vi "Check Target Internet Connection.vi"(8 "Error In":errorcluster, 11 "Install LV Data":T1={"SSH Session"=refnum, "Status Log"="", "Detailed Log"="", "Credentials"={"Hostname or IP"="192.168.7.2", "Username"="root", "Password"=""}, "Target Info"={"OS Version"="", "CPU"="", "Systemd Version"="", "Internet Access"=FALSE, "Device Type"=""}, "Reboot Required?"=FALSE}) -> (0 "Error Out":errorcluster, 3 "Install LV Data":T1={"SSH Session"=refnum, "Status Log"="", "Detailed Log"="", "Credentials"={"Hostname or IP"="192.168.7.2", "Username"="root", "Password"=""}, "Target Info"={"OS Version"="", "CPU"="", "Systemd Version"="", "Internet Access"=FALSE, "Device Type"=""}, "Reboot Required?"=FALSE})   [LabVIEW 2014, in "LMH-LINX.lvlib"]
uses:
  LMH-LINX.lvlib
  Install LV Data.ctl
  C:/github/makerhub/LINX/LabVIEW/vi.lib/MakerHub/LINX/Resources/Renci.SshNet.dll
  Resources/Renci.SshNet.dll
  Target Info.ctl
  <vilib>/regexp/Match Regular Expression.xnode
panel:
  out "Internet Connection?":bool
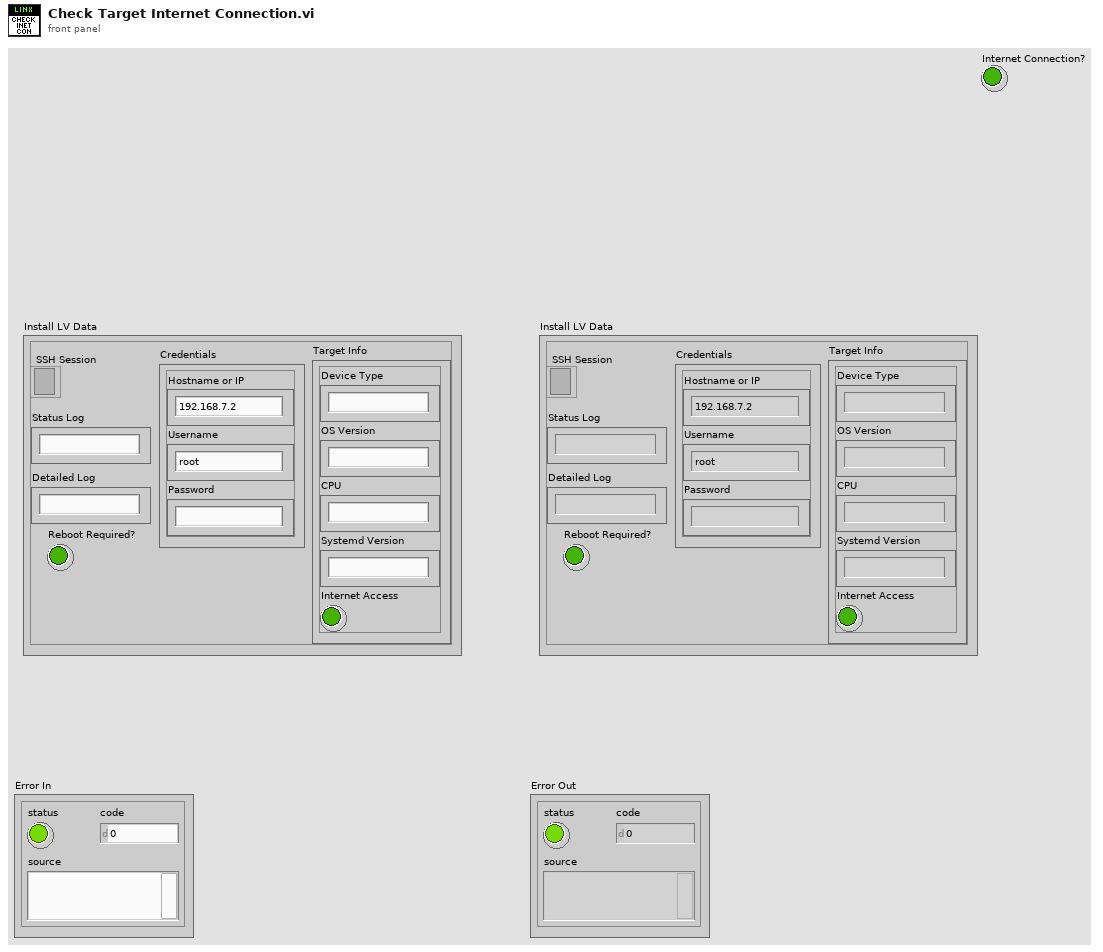
[diagram p1: front panel]
types:
  T1 = typedef "LMH-LINX.lvlib/Install LV Data.ctl" = cluster{"SSH Session":refnum<k24>, "Status Log":string, "Detailed Log":string, "Credentials":cluster{"Hostname or IP":string, "Username":string, "Password":string}, "Target Info":T2, "Reboot Required?":bool}
  T2 = typedef "LMH-LINX.lvlib/Target Info.ctl" = cluster{"OS Version":string, "CPU":string, "Systemd Version":string, "Internet Access":bool, "Device Type":string}
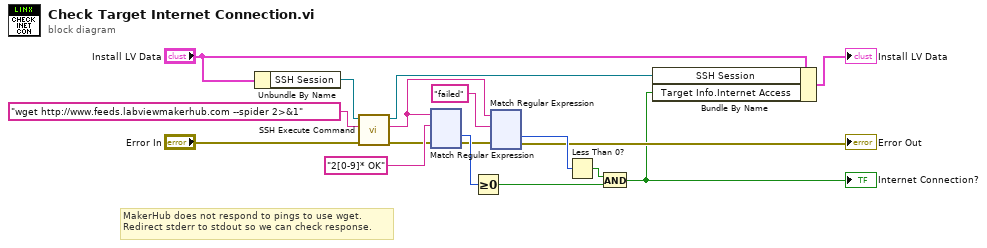
[diagram p0: block diagram]
diagram:
  # "MakerHub does not respond to pings to use wget.\nRedirect stderr to stdout so we can check response."
  n1 = Unbundle By Name("Install LV Data") -> ("SSH Session"=w16:refnum<k24>)
  n2 = call "SSH Execute Command.vi"("Error In"="Error In", "Command"="wget http://www.feeds.labviewmakerhub.com --spider 2>&1", "SSH Session"=w16) -> ("Error Out"=w4:errorcluster, "Std Out"=w6:string, "SSH Session"=w14:refnum<k24>)  [unwired: 6 in]
  n3 = xnode "Match Regular Expression"("input string"=w6, "regular expression"="2[0-9]* OK", "error in"=w4) -> ("offset past match"=w11:i32, "error out"=w5:errorcluster)  [unwired: 3 in, 3 out]
  n4 = Greater Or Equal To 0?(x=w11) -> (x >= 0?=w8:bool)
  n5 = xnode "Match Regular Expression"("input string"=w6, "regular expression"="failed", "error in"=w5) -> ("offset past match"=w9:i32, "error out"=→"Error Out":errorcluster)  [unwired: 3 in, 3 out]
  n6 = Less Than 0?(x=w9) -> (x < 0?=w7:bool)
  n7 = And(x=w7, y=w8) -> (x .and. y?=w2:bool)
  "Internet Connection?" <- w2
  n8 = Bundle By Name(cluster="Install LV Data", "SSH Session"=w14, "Target Info.Internet Access"=w2) -> (→"Install LV Data":T1)
